vi "MESADCLogin.vi"(8 "barcode":string, 9 "电脑名":string, 10 "簇":T1={"工号"="2300013", "站别"="F1", "站名"="写信息", "表名称"="test", "工单号"="85255", "条码"="EC82637770B0", "路径"="", "是否连接"=0, "电脑名"=""}) -> (0 "布尔":bool, 2 "message":string)   [LabVIEW 2014]
uses:
  dll/MESControldll.dll
panel:
  out "PointGroup 2":string
  out "PointName 2":string
  out "userid 2":string
  out "POnum 1":i32
  out "result":i32
  out "错误输出":errorcluster
  in  "错误输入（无错误）":errorcluster
  # "2300013"
  # "447BBBCDFA60"
  # "MES:CHECK OK"
  # "1001594"
  # "0是代表OK，-1代表NG"
  # "计算机名"
  # "447BBBA1A0D0"
  # "MES:SN [EC82637A4880] \n不允许此测试 [F2]! 当前节点 [F1]"
  # "1001608"
  # "EC8263799B78\nSay{FAIL.wav}请维护规程 [整机维修] 的测试代码!"
  # "85353"
  # "21080"
  # "2300013\n18132D7F0694\n85174\nF6信息核对"
  # "2300013\n447BBBA12C40\n85197\nF6接口测试"
  # "2300013\nEC82637770B0\n85255\nF1信息写入"
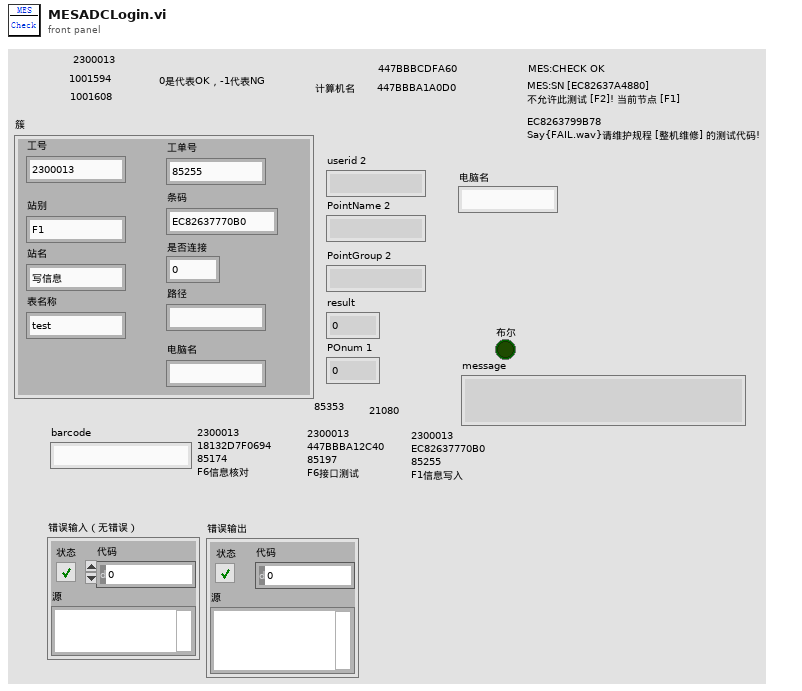
[diagram p1: front panel]
types:
  T1 = cluster{"工号":string, "站别":string, "站名":string, "表名称":string, "工单号":string, "条码":string, "路径":string, "是否连接":i32, "电脑名":string}
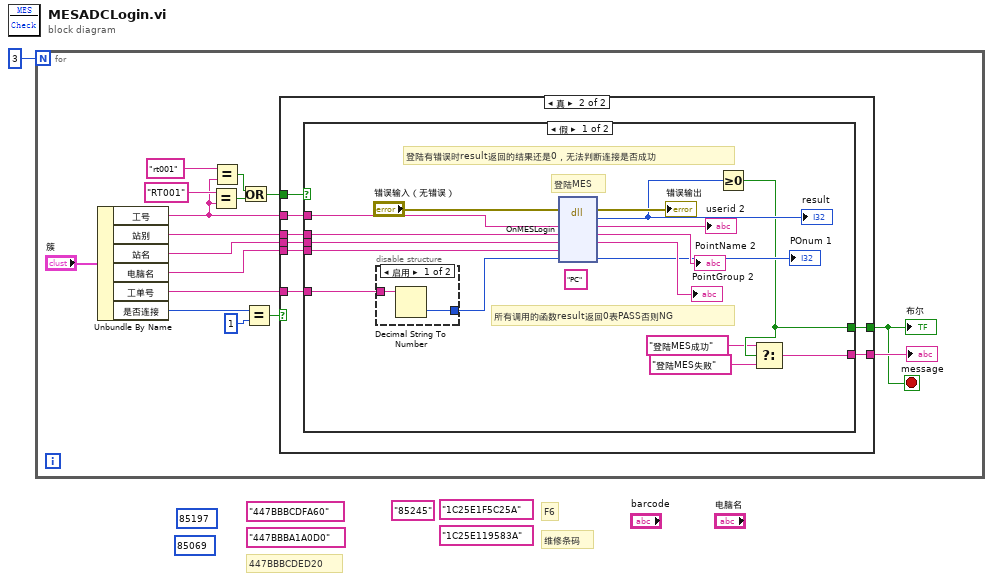
[diagram p0: block diagram]
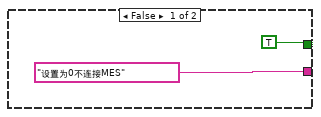
[diagram p2: hidden frame]
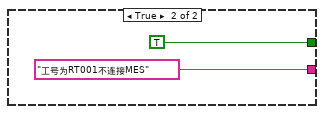
[diagram p4: hidden frame]
diagram:
  (unwired) 85069 ("EquipID")
  (unwired) "447BBBCDFA60"
  (unwired) "1C25E119583A"
  (unwired) "1C25E1F5C25A"
  (unwired) 85197 ("EquipID")
  (unwired) "85245"
  (unwired) "447BBBA1A0D0"
  # "447BBBCDED20"
  # "维修条码"
  # "F6"
  n1 = for {
    N: 3 -> [_]
    stop <- w9 stop-if-true
    n2 = Unbundle By Name("簇") -> ("工号"=w7:string, "站别"=w6:string, "站名"=w5:string, "电脑名"=w4:string, "工单号"=w3:string, "是否连接"=w2:i32)
    n3 = Equal?(x="RT001", y=w7) -> (x = y?=w11:bool)
    n4 = Equal?(x="rt001", y=w7) -> (x = y?=w12:bool)
    n5 = Or(x=w12, y=w11) -> (x .or. y?=w10:bool)
    n6 = Equal?(x=w2, y=1 ("偏移量(0)")) -> (x = y?=w16:bool)
    n7 = case shown="真" w16 {
      tunnel: [TRUE w27] -> w9
      tunnel: ["设置为0不连接MES" ("key") w26] -> w17
      tunnel: w7 -> [_ w25]
      tunnel: w6 -> [_ w24]
      tunnel: w10 -> [_ w23]
      tunnel: w5 -> [_ w22]
      tunnel: w4 -> [_ w21]
      tunnel: w3 -> [_ w20]
      frame False {
      }
      frame True {
        n8 = case shown="假" w23 {
          tunnel: [w34 TRUE] -> w27
          tunnel: [w33 "工号为RT001不连接MES" ("key")] -> w26
          tunnel: w25 -> [w39 _]
          tunnel: w24 -> [w38 _]
          tunnel: w22 -> [w30 _]
          tunnel: w21 -> [w29 _]
          tunnel: w20 -> [w28 _]
          frame False {
            (unwired) "PC" ("PointPlace")
            # "登陆MES"
            # "登陆有错误时result返回的结果还是0，无法判断连接是否成功"
            # "所有调用的函数result返回0表PASS否则NG"
            n9 = disable-structure shown="启用" {
              disable-tunnel: w28 -> [w46 _]
              disable-tunnel: [w45 _] -> w35
              frame Enabled {
                n10 = Decimal String To Number(string=w46) -> (number=w45:i32)  [unwired: 2 in, 1 out]
              }
              frame Disabled {
              }
            }
            n11 = dll-call lib="PTH2@abs Eli产品文件MESMESMESdllMESControldll.dll" fn="OnMESLogin"(error in="错误输入（无错误）", "userid"=w39, "PointName"=w38, "PointGroup"=w30, "PointPlace"=w29, "EquipID"=w35) -> (error out=→"错误输出":errorcluster, "result"=w36:i32, "userid"=→"userid 2":string, "PointName"=→"PointName 2":string, "PointGroup"=→"PointGroup 2":string, "EquipID"=→"POnum 1":i32)  [unwired: 3 in, 1 out]
            "result" <- w36
            n12 = Greater Or Equal To 0?(x=w36) -> (x >= 0?=w34:bool)
            n13 = Select(t="登陆MES成功", s=w34, f="登陆MES失败") -> (s? t:f=w33:string)
          }
          frame True {
          }
        }
      }
    }
    "布尔" <- w9
    "message" <- w17
  }
